vi "Error Monitor.vi"(6 "Error Codes to Ignore":i32[](array[numeric]), 8 "error in":errorcluster, 10 "State":string, 11 "QDMH in":refnum<class "QDMH.lvclass">) -> (0 "error out":errorcluster, 3 "QDMH out":refnum<class "QDMH.lvclass">)   [LabVIEW 2023, in "QDMH.lvlib" / "QDMH.lvclass"]
uses:
  QDMH.lvclass
  Custom Controls/QDMH Message.ctl
  Private/Enqueue Bundled Element.vi
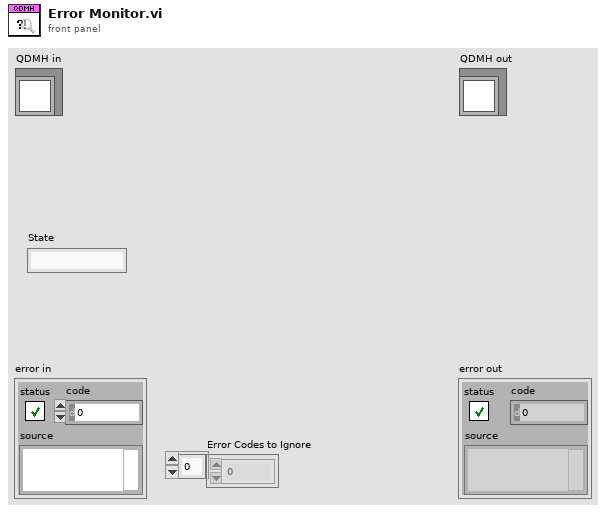
[diagram p1: front panel]
types:
  T1 = typedef "QDMH.lvlib/QDMH.lvclass/QDMH Message.ctl" = cluster{"State":string, "Data":variant}
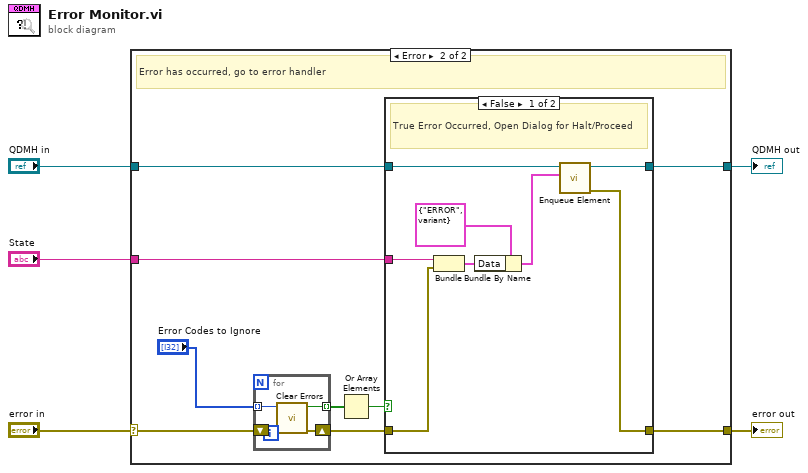
[diagram p0: block diagram]
diagram:
  n1 = case shown="Error" "error in" {
    selector: "error in" -> [w6 w16]
    tunnel: [w6 w11] -> w4
    tunnel: [w7 w9] -> w2
    tunnel: "QDMH in" -> [w7 w10]
    tunnel: "State" -> [_ w8]
    frame No Error {
      # "No Error occurred, proceed to the next state"
    }
    frame Error {
      # "Error has occurred, go to error handler"
      n2 = for {
        tunnel: "Error Codes to Ignore" -> [w18] mode=indexing
        shift-right: [w19] -> w15
        shift-left: w16 -> [w20]
        tunnel: [w17] -> w13 mode=indexing
        n3 = call <vilib>:"Clear Errors.vi"("error in (no error)"=w20, "specific error code to clear (0: all)"=w18) -> ("error out"=w19:errorcluster, "specific error cleared?"=w17:bool)  [unwired: 4 in]
      }
      n4 = Or Array Elements(Boolean array=w13) -> (logical OR=w12:bool)
      n5 = case shown="False" w12 {
        tunnel: w15 -> [w22 w30]
        tunnel: [w26 w30] -> w11
        tunnel: w10 -> [w28 w29]
        tunnel: [w27 w29] -> w9
        tunnel: w8 -> [w21 _]
        frame False {
          # "True Error Occurred, Open Dialog for Halt/Proceed"
          n6 = Bundle("State"=w21, "error IO"=w22) -> (w23:cluster{"State":string, "error IO":errorcluster})  [unwired: 1 in]
          n7 = Bundle By Name(cluster=T1 {"State"="ERROR", "Data"=variant} ("Message"), "Data"=w23) -> (w24:T1)
          n8 = call-poly "Enqueue Element.vi"("element"=w24, "QDMH in"=w28) -> ("error out"=w26:errorcluster, "QDMH out"=w27:refnum<class "QDMH.lvclass">)  [unwired: 8 in]
        }
        frame True {
          # "Error that occurred was ignored, proceed to next step"
        }
      }
    }
  }
  "error out" <- w4
  "QDMH out" <- w2
